vi "FTW-ProjectItem-GetItemInfo.vi"(0 "ProjectItem":refnum<vi>, 11 "error in":errorcluster) -> (4 "ProjectItem out":refnum<vi>, 6 "ItemID":string, 8 "Display Name":string, 10 "Item Type GUID":string, 15 "error out":errorcluster)   [LabVIEW 2012]
panel:
  # "Inputs"
  # "Outputs"
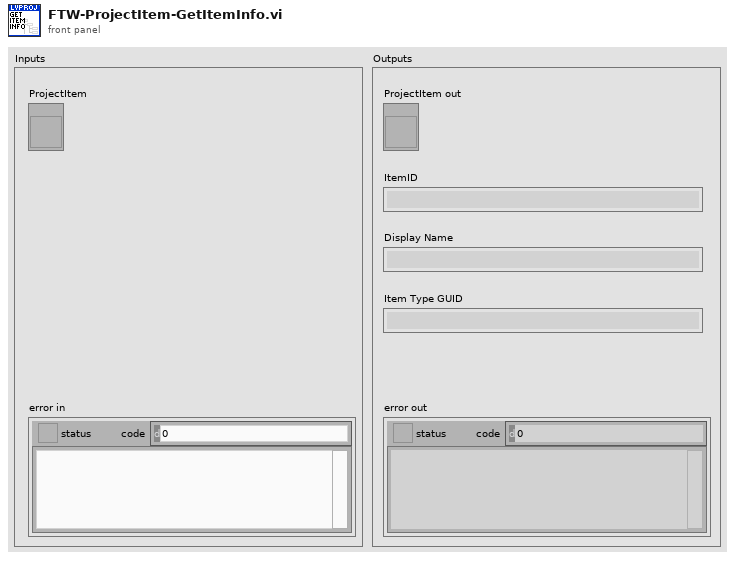
[diagram p1: front panel]
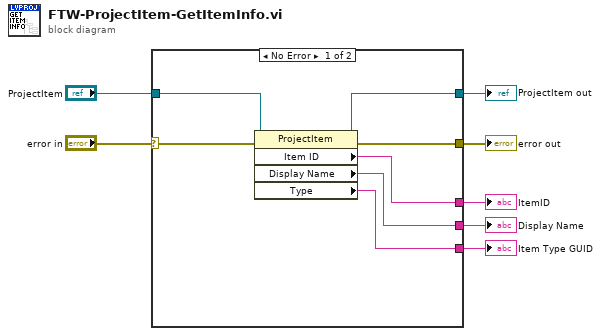
[diagram p0: block diagram]
diagram:
  n1 = case shown="No Error" "error in" {
    selector: "error in" -> [w13 w16]
    tunnel: [w12 w16] -> w7
    tunnel: "ProjectItem" -> [w14 w15]
    tunnel: [w11 _] -> w4
    tunnel: [w10 _] -> w3
    tunnel: [w8 _] -> w2
    tunnel: [w9 w15] -> w1
    frame No Error {
      n2 = property class="ProjectItem"(reference=w14, error in=w13) -> (reference out=w9:refnum<vi>, error out=w12:errorcluster, "Item ID"=w8:string, "Display Name"=w11:string, "Type"=w10:string)
    }
    frame Error {
    }
  }
  "error out" <- w7
  "Display Name" <- w4
  "Item Type GUID" <- w3
  "ItemID" <- w2
  "ProjectItem out" <- w1
